vi "csmdoc_export_VI_description.vi"(7 "NOTE-Map":variant, 8 "error in (no error)":errorcluster, 11 "Path":path) -> (0 "error out":errorcluster, 3 "concatenated string":string)   [LabVIEW 2017, in "csmdoc.lvlib"]
uses:
  csmdoc.lvlib
  Communicable State Machine.lvlib
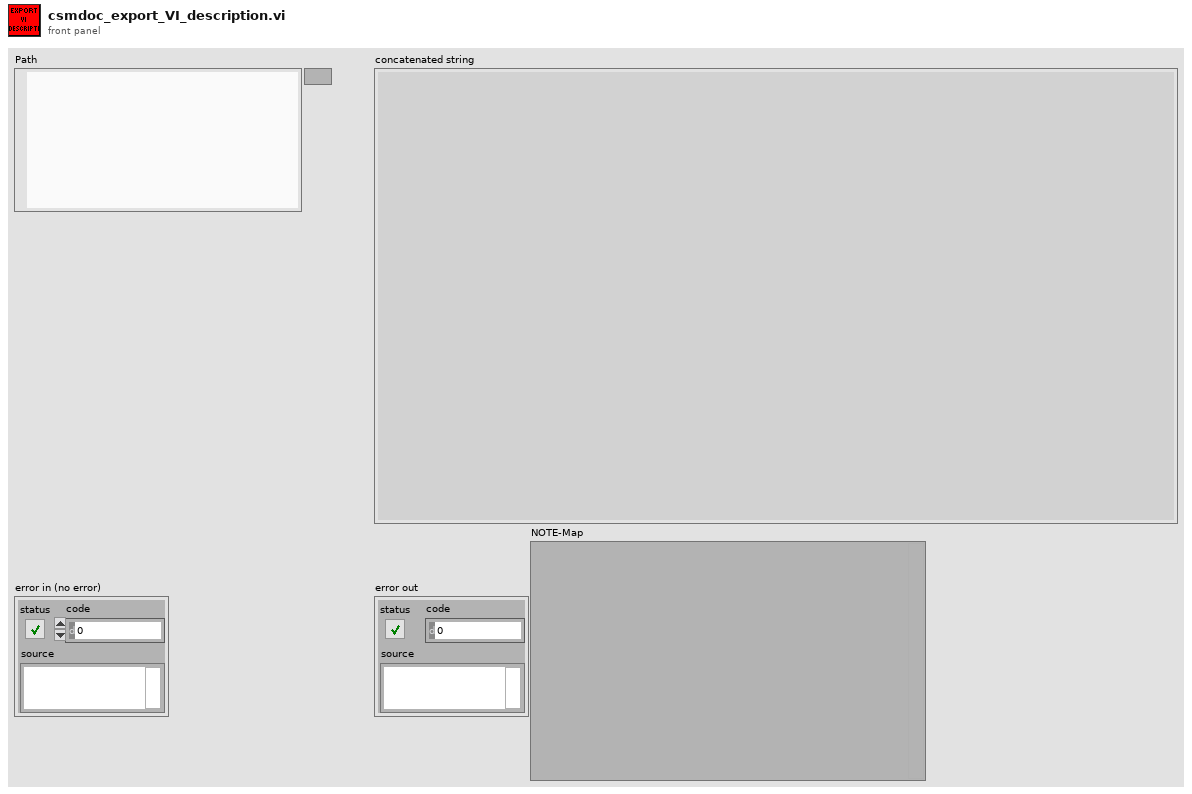
[diagram p1: front panel]
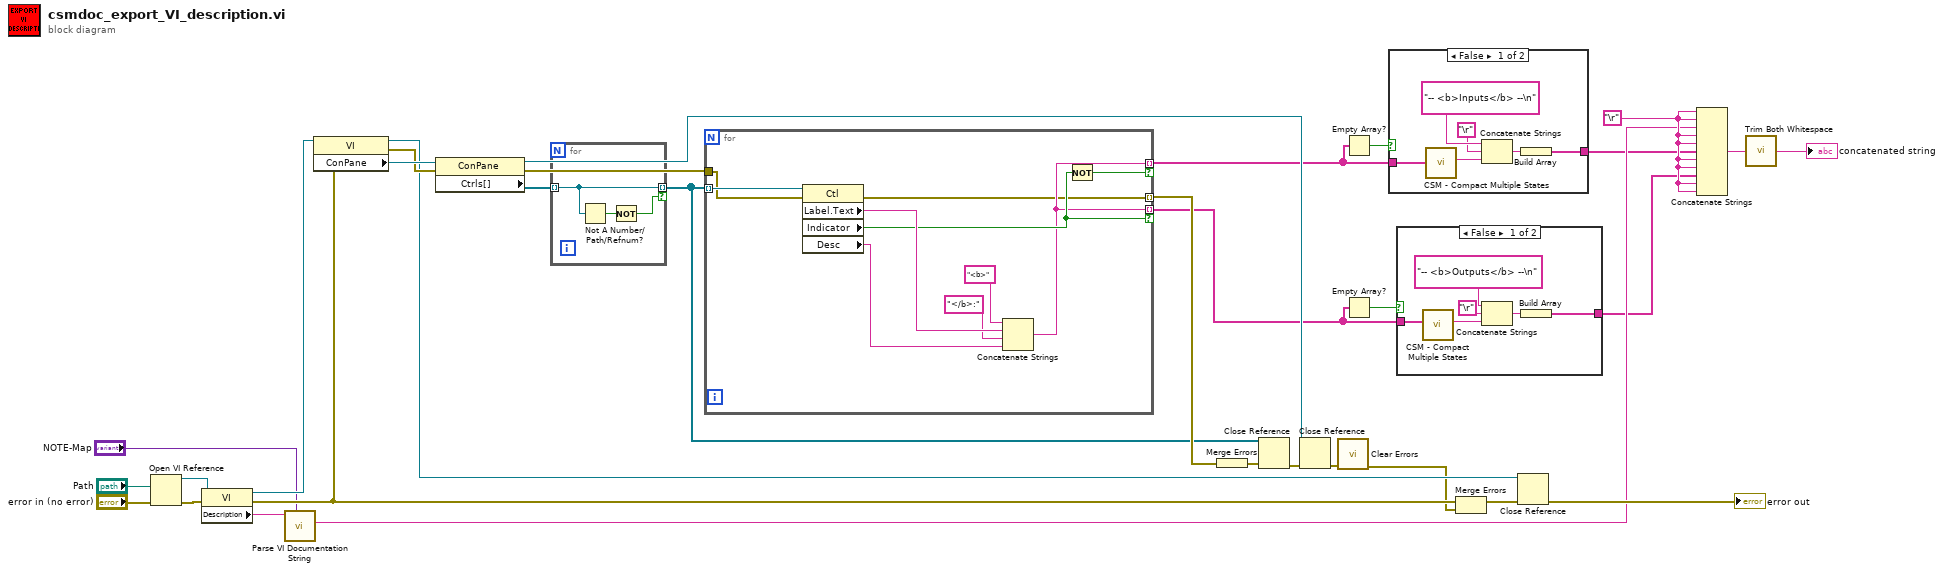
[diagram p0: block diagram]
diagram:
  w21 = "\r"
  n1 = Open VI Reference(vi path="Path", error in (no error)="error in (no error)") -> (vi reference=w31:refnum<vi>, error out=w32:errorcluster)  [unwired: 4 in]
  n2 = property class="VI"(reference=w31, error in=w32) -> (reference out=w30:refnum<vi>, error out=w20:errorcluster, "Description"=w9:string)
  n3 = call "Parse VI Documentation String.vi"("NOTE-Map"="NOTE-Map", "Documentation"=w9) -> ("Core Doc"=w8:string)  [unwired: 6 in, 3 out]
  n4 = property class="VI"(reference=w30, error in=w20) -> (reference out=w22:refnum<vi>, error out=w28:errorcluster, "ConPane"=w29:refnum<vi>)
  n5 = property class="ConPane"(reference=w29, error in=w28) -> (reference out=w23:refnum<vi>, error out=w26:errorcluster, "Ctrls[]"=w11:refnum<vi>[])
  n6 = for {
    tunnel: w11 -> [w35] mode=indexing
    tunnel: [w35] -> w10 mode=indexing if=w33
    n7 = Not A Number/Path/Refnum?(number/path/refnum=w35) -> (NaN/Path/Refnum?=w34:bool)
    n8 = Not(x=w34) -> (.not. x?=w33:bool)
  }
  n9 = for {
    tunnel: w10 -> [w45] mode=indexing
    tunnel: [w41] -> w4 mode=indexing if=w42
    tunnel: [w41] -> w5 mode=indexing if=w43
    tunnel: w26 -> [w39]
    tunnel: [w38] -> w25 mode=indexing
    n10 = property class="Ctl"(reference=w45, error in=w39) -> (error out=w38:errorcluster, "Label.Text"=w44:string, "Indicator"=w43:bool, "Desc"=w36:string)  [unwired: 1 out]
    n11 = Concatenate Strings("<b>" ("string"), w44, "</b>:" ("string"), w36) -> (w41:string)
    n12 = Not(x=w43) -> (.not. x?=w42:bool)
  }
  n13 = Merge Errors(w25) -> (w24:errorcluster)
  n14 = Close Reference(reference=w10, error in (no error)=w24) -> (error out=w27:errorcluster)
  n15 = Close Reference(reference=w23, error in (no error)=w27) -> (error out=w19:errorcluster)
  n16 = call <vilib>:"Clear Errors.vi"("error in (no error)"=w19) -> ("error out"=w13:errorcluster)  [unwired: 5 in, 1 out]
  n17 = Empty Array?(array=w4) -> (empty?=w3:bool)
  n18 = Empty Array?(array=w5) -> (empty?=w2:bool)
  n19 = case shown="False" w3 {
    tunnel: [w47 _] -> w6
    tunnel: w4 -> [w46 _]
    frame False {
      n20 = call "CSM - Compact Multiple States.vi"("Multiple States"=w46) -> ("States"=w51:string)  [unwired: 9 in]
      n21 = Concatenate Strings("-- <b>Inputs</b> --\n" ("string"), "\r", w51) -> (w49:string)
      n22 = Build Array(w49) -> (w47:string[])
    }
    frame True {
    }
  }
  n23 = case shown="False" w2 {
    tunnel: [w54 _] -> w7
    tunnel: w5 -> [w52 _]
    frame False {
      n24 = call "CSM - Compact Multiple States.vi"("Multiple States"=w52) -> ("States"=w57:string)  [unwired: 9 in]
      n25 = Concatenate Strings("-- <b>Outputs</b> --\n" ("string"), "\r", w57) -> (w55:string)
      n26 = Build Array(w55) -> (w54:string[])
    }
    frame True {
    }
  }
  n27 = Merge Errors(w20, w13) -> (w18:errorcluster)
  n28 = Close Reference(reference=w22, error in (no error)=w18) -> (error out=→"error out":errorcluster)
  n29 = Concatenate Strings(w21, w21, w8, w21, w21, w6, w21, w21, w7, w21, w21) -> (w16:string)
  n30 = call "Trim Both Whitespace.vi"("string"=w16) -> ("trimmed string"=→"concatenated string":string)  [unwired: 1 in]
